vi "LV_Img_transfer.vi"() -> ()   [LabVIEW 2020]
panel:
  out "Elapsed time [ms]":u32
  out "standard error from Python":string
  in  "h":i32=10 min=1 max=5000 step=1
  in  "w":i32=1 min=1 max=5000 step=1
  out "standard output from Python":string
  out "error out":errorcluster
  out "Path to Python script":path
  # "For only image transfer \n(not converting image)"
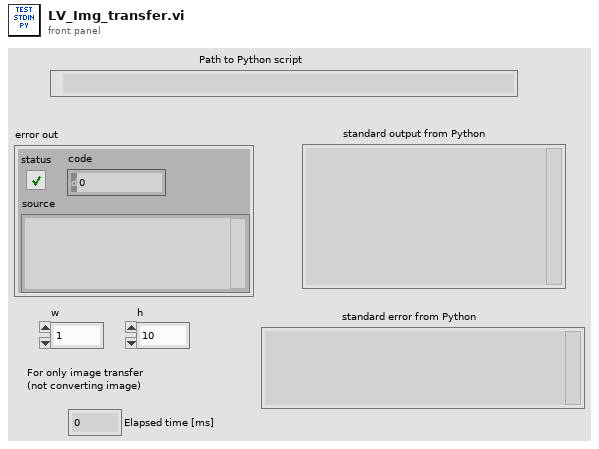
[diagram p1: front panel]
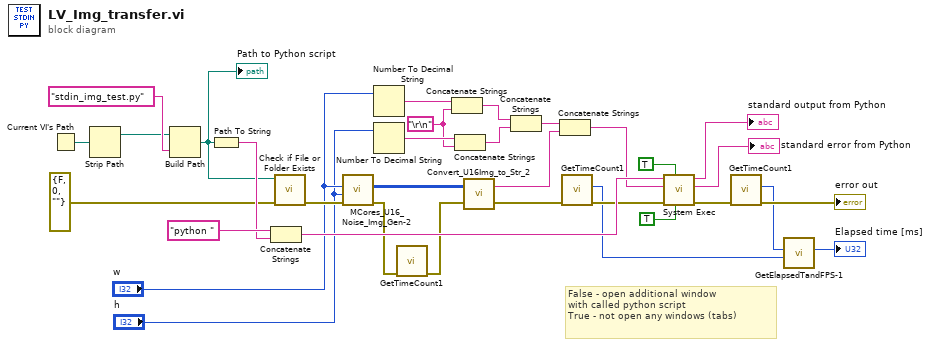
[diagram p0: block diagram]
diagram:
  w16 = "\r\n"
  # "False - open additional window\nwith called python script\nTrue - not open any windows (tabs)"
  n1 = Current VI's Path() -> (path=w33:path)
  n2 = Strip Path(path=w33) -> (stripped path=w27:path)  [unwired: 1 out]
  n3 = Build Path(base path=w27, name or relative path="stdin_img_test.py" ("string")) -> (appended path=w25:path)
  "Path to Python script" <- w25
  n4 = Path To String(path=w25) -> (string=w28:string)
  n5 = Concatenate Strings("python " ("command line"), w28) -> (w31:string)
  n6 = call <vilib>:"Check if File or Folder Exists.vi"("error in (no error)"=errorcluster {"status"=FALSE, "code"=0, "source"=""}, "path"=w25) -> ("error out"=w22:errorcluster)  [unwired: 7 in, 2 out]
  n7 = call "MCores_U16_Noise_Img_Gen-2.vi"("error IN"=w22, "[IN] Width"="h", "[IN] Height"="w") -> ("error OUT"=w9:errorcluster, "[OUT] U16 Pixel Img"=w21:u16[][])  [unwired: 7 in]
  n8 = Number To Decimal String(number="w") -> (decimal integer string=w18:string)  [unwired: 1 in]
  n9 = Number To Decimal String(number="h") -> (decimal integer string=w17:string)  [unwired: 1 in]
  n10 = call "GetTimeCount1.vi"("error IN"=w9) -> ("error OUT"=w8:errorcluster)  [unwired: 9 in, 1 out]
  n11 = Concatenate Strings(w18, w16) -> (w15:string)
  n12 = Concatenate Strings(w17, w16) -> (w14:string)
  n13 = call "Convert_U16Img_to_Str_2.vi"("error IN"=w8, "[IN] U16 Pixel Img"=w21) -> ("error OUT"=w4:errorcluster, "[OUT] Raw string"=w12:string)
  n14 = Concatenate Strings(w15, w14) -> (w13:string)
  n15 = Concatenate Strings(w13, w12) -> (w11:string)
  n16 = call "GetTimeCount1.vi"("error IN"=w4) -> ("error OUT"=w3:errorcluster, "[OUT] Timer Count"=w2:u32)  [unwired: 9 in]
  n17 = call <vilib>:"System Exec.vi"("run minimized? (F)"=TRUE, "wait until completion? (T)"=TRUE, "error in (no error)"=w3, "standard input"=w11, "command line"=w31) -> ("error out"=w7:errorcluster, "standard error"=→"standard error from Python":string, "standard output"=→"standard output from Python":string)  [unwired: 3 in, 1 out]
  n18 = call "GetTimeCount1.vi"("error IN"=w7) -> ("error OUT"=→"error out":errorcluster, "[OUT] Timer Count"=w1:u32)  [unwired: 9 in]
  n19 = call "GetElapsedTandFPS-1.vi"("[IN] Timer Count Before ALL [ms]"=w2, "[IN] Timer Count After ALL [ms]"=w1) -> ("[OUT] Elapsed time [ms]"=→"Elapsed time [ms]":u32)  [unwired: 3 in, 2 out]
